vi "VSET.vi"(8 "error in (no error)":errorcluster, 9 "Value (0-30)":dbl min=0.0 max=30.0, 10 "Channel in":T1, 11 "refnum in":T2) -> (0 "error out":errorcluster, 2 "Channel out":T1, 3 "refnum out":T2, 4 "question out":string)   [LabVIEW 2021, in "Korad KA3305P.lvlib"]
uses:
  Korad KA3305P.lvlib
  Channels.ctl
  Reference.ctl
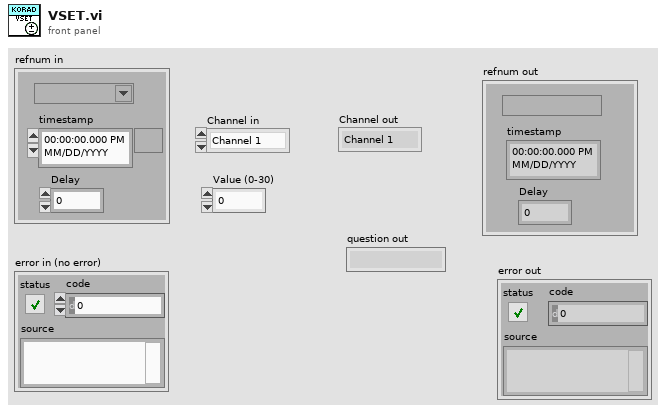
[diagram p1: front panel]
types:
  T1 = typedef "Korad KA3305P.lvlib/Channels.ctl" = enum16{"Channel 1", "Channel 2"}
  T2 = typedef "Korad KA3305P.lvlib/Reference.ctl" = cluster{"refnum":refnum<visa-resource-name>, "timestamp":timestamp, "Delay":dbl}
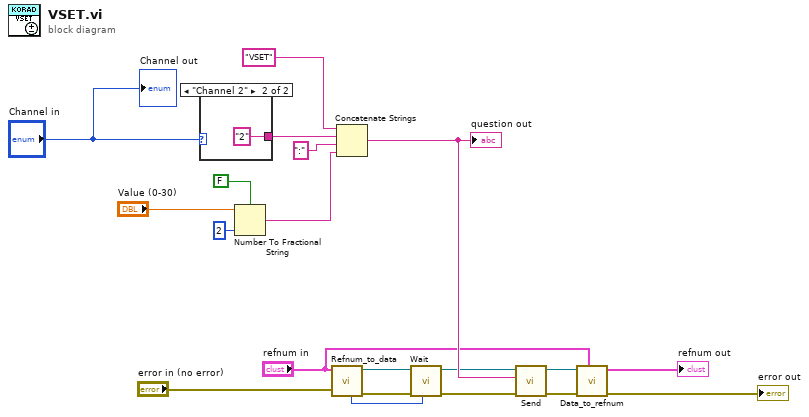
[diagram p0: block diagram]
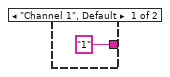
[diagram p2: hidden frame]
diagram:
  n1 = case shown="\"Channel 2\"" "Channel in" {
    tunnel: ["1" "2"] -> w19
    frame "Channel 1", Default {
    }
    frame "Channel 2" {
    }
  }
  n2 = Number To Fractional String(use system decimal point (T)=FALSE, number="Value (0-30)", precision (6)=i16 2) -> (F-format string=w15:string)  [unwired: 1 in]
  n3 = call "Refnum_to_data.vi"("error in (no error)"="error in (no error)", "refnum in"="refnum in") -> ("error out"=w8:errorcluster, "DAQ refnum out"=w7:refnum<visa-resource-name>, "delay out"=w6:u32)  [unwired: 7 in]
  n4 = Concatenate Strings("VSET" ("string"), w19, ":" ("string"), w15) -> (w13:string)
  "question out" <- w13
  n5 = call "Wait.vi"("milliseconds to wait"=w6, "error in (no error)"=w8, "refnum in"=w7) -> ("error out"=w12:errorcluster, "refnum out"=w10:refnum<visa-resource-name>)  [unwired: 7 in]
  n6 = call "Send.vi"("error in (no error)"=w12, "data"=w13, "refnum in"=w10) -> ("error out"=w9:errorcluster, "refnum out"=w4:refnum<visa-resource-name>)  [unwired: 7 in]
  n7 = call "Data_to_refnum.vi"("refnum in"="refnum in", "error in (no error)"=w9, "DAQ refnum in"=w4) -> ("error out"=→"error out":errorcluster, "refnum out"=→"refnum out":T2)  [unwired: 7 in]
  "Channel out" <- "Channel in"
